vi "Update SD Channels.vi"(7 "Type":T2, 8 "error in (no error)":errorcluster, 9 "Channel Names":string[](array[string]), 10 "Node Ptr In":T1 format="%.0x", 11 "SD Module in":refnum<class "SD Module.lvclass">) -> (0 "error out":errorcluster, 2 "Node Ptr Out":T1 format="%.0x", 3 "SD Module out":refnum<class "SD Module.lvclass">)   [LabVIEW 2017, in "Modules.lvlib" / "SD Module.lvclass"]
uses:
  SD Module.lvclass
  C:/Users/dbuck/Documents/GitHub/Scan-Engine-Custom-Device-Classes/Source/RSI Module/RSI Module.lvclass
  <vilib>/NI Veristand/Custom Device API/Custom Device Channel Type.ctl
  <vilib>/NI Veristand/Custom Device API/Custom Device Item Ref.ctl
  <vilib>/NI Veristand/Custom Device API/Custom Device Channel.ctl
  RSI Module/Class Property Strings.vi
  RSI Module/Channel GUIDs.vi
  RSI Module/RSI Module.lvclass
  <vilib>/NI Veristand/Custom Device API/Custom Device API.lvlib
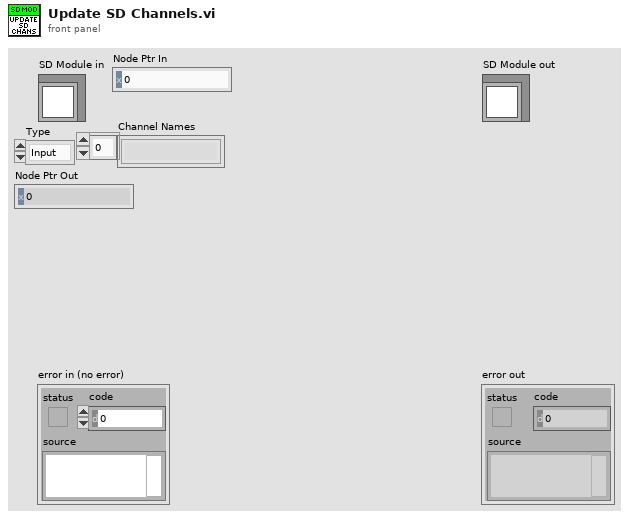
[diagram p1: front panel]
types:
  T1 = typedef "Custom Device API.lvlib/Custom Device Item Ref.ctl" = u64
  T2 = typedef "Custom Device API.lvlib/Custom Device Channel Type.ctl" = enum16{"Input", "Output"}
  T3 = typedef "Custom Device API.lvlib/Custom Device Channel.ctl" = cluster{"Type":T2, "Units":string, "Default Value":dbl, "Faultable":bool, "Scalable":bool}
  T4 = typedef "Modules.lvlib/RSI Module.lvclass/Channels.ctl" = cluster{"# Input Channels":i32, "# Output Channels":i32, "Channel Type":T5, "Units":string}
  T5 = typedef "Modules.lvlib/RSI Module.lvclass/Channel Type.ctl" = enum16{"Analog", "Digital"}
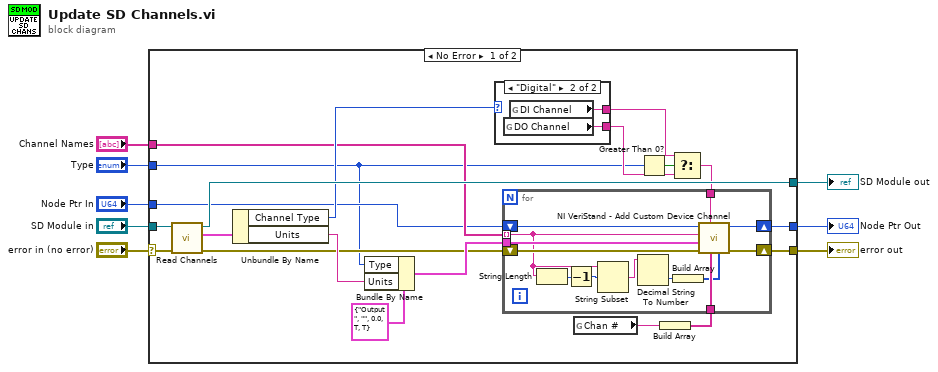
[diagram p0: block diagram]
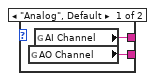
[diagram p2: hidden frame]
diagram:
  n1 = case shown="No Error" "error in (no error)" {
    selector: "error in (no error)" -> [w13 w48]
    tunnel: [w12 w48] -> w7
    tunnel: [w27 w47] -> w5
    tunnel: "SD Module in" -> [w28 w47]
    tunnel: "Type" -> [w10 _]
    tunnel: "Channel Names" -> [w15 _]
    tunnel: "Node Ptr In" -> [w11 w46]
    tunnel: [w9 w46] -> w1
    frame No Error {
      n2 = call "Read Channels.vi"("error in (no error)"=w13, "RSI Module in"=w28) -> ("error out"=w14:errorcluster, "Channels"=w16:T4, "RSI Module out"=w27:refnum<class "SD Module.lvclass">)  [unwired: 7 in]
      n3 = Unbundle By Name(w16) -> ("Channel Type"=w26:T5, "Units"=w18:string)
      n4 = Bundle By Name(cluster=T3 {"Type"=enum."Output", "Units"="", "Default Value"=0.0, "Faultable"=TRUE, "Scalable"=TRUE} ("Channel"), "Type"=w10, "Units"=w18) -> (w19:T3)
      n5 = case shown="\"Digital\"" w26 {
        tunnel: [w30 w32] -> w23
        tunnel: [w29 w31] -> w24
        frame "Analog", Default {
          n6 = global read "Channel GUIDs.vi" "AO Channel"() -> (w29:string)
          n7 = global read "Channel GUIDs.vi" "AI Channel"() -> (w30:string)
        }
        frame "Digital" {
          n8 = global read "Channel GUIDs.vi" "DO Channel"() -> (w31:string)
          n9 = global read "Channel GUIDs.vi" "DI Channel"() -> (w32:string)
        }
      }
      n10 = global read "Class Property Strings.vi" "Chan #"() -> (w20:string)
      n11 = Greater Than 0?(x=w10) -> (x > 0?=w22:bool)
      n12 = Build Array(w20) -> (w21:string[])
      n13 = Select(t=w23, s=w22, f=w24) -> (s? t:f=w25:string)
      n14 = for {
        tunnel: w15 -> [w36] mode=indexing
        shift-right: [w41] -> w12
        shift-left: w14 -> [w45]
        tunnel: w19 -> [w44]
        shift-right: [w42] -> w9
        shift-left: w11 -> [w43]
        tunnel: w21 -> [w40]
        tunnel: w25 -> [w33]
        n15 = String Length(string=w36) -> (length=w35:i32)
        n16 = Decrement(x=w35) -> (x-1=w34:i32)
        n17 = String Subset(string=w36, offset (0)=w34) -> (substring=w38:string)  [unwired: 1 in]
        n18 = Decimal String To Number(string=w38) -> (number=w37:i32)  [unwired: 2 in, 1 out]
        n19 = Build Array(w37) -> (w39:i32[])
        n20 = call <vilib>:"NI VeriStand - Add Custom Device Channel.vi"("Property Values"=w39, "Property names"=w40, "GUID (Default Channel)"=w33, "error in (no error)"=w45, "Channel"=w44, "Channel Name"=w36, "Parent Ref in"=w43) -> ("error out"=w41:errorcluster, "Parent Ref out"=w42:T1)  [unwired: 1 in, 2 out]
      }
    }
    frame Error {
    }
  }
  "error out" <- w7
  "SD Module out" <- w5
  "Node Ptr Out" <- w1
